vi "SendNetworkMsg.vi"(0 "reference in":refnum<class "MessageInterface.lvclass">, 1 "receiver process":string, 2 "receiver host":string, 3 "receiver port (0)":u16, 5 "name":string, 7 "value":string, 9 "timeout (25000 ms)":i32=25000, 11 "error in (no error)":errorcluster) -> (4 "reference out":refnum<class "MessageInterface.lvclass">, 10 "timed out?":bool, 15 "error out":errorcluster)   [LabVIEW 2019, in "MessageInterface.lvclass"]
uses:
  MessageInterface.lvclass
  <vilib>/Utility/error.llb/Error Cluster From Error Code.vi
  <vilib>/ErrorRing/Error Ring.xnode
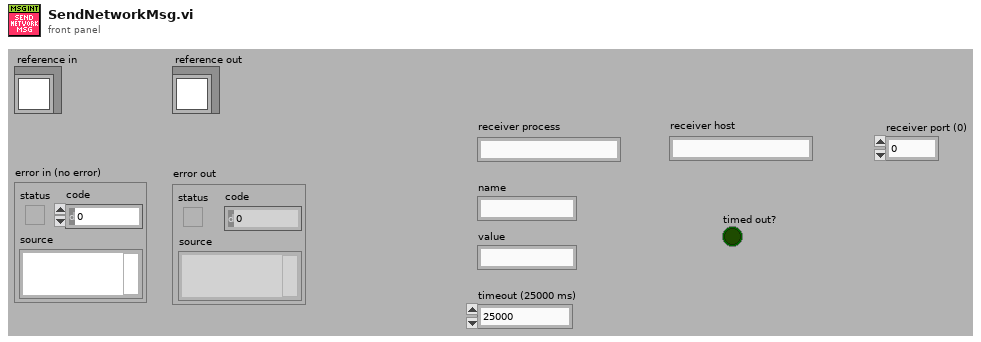
[diagram p1: front panel]
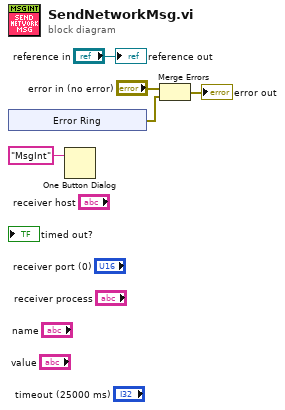
[diagram p0: block diagram]
diagram:
  n1 = xnode "Error Ring"() -> ("error out"=w3:errorcluster)
  n2 = One Button Dialog(message="MsgInt") -> ()  [unwired: 1 in, 1 out]
  n3 = Merge Errors("error in (no error)", w3) -> (→"error out":errorcluster)
  "reference out" <- "reference in"
